vi "ExampleAppAssembler.vi"() -> ()   [LabVIEW 2017]
uses:
  <vilib>/ActorFramework/Message Enqueuer/Message Priority.ctl
  <vilib>/gpm_packages/@cs/mva-viewable/Source/IViewable/IViewable/View Position Enum.ctl
  ViewModel/ViewModel/Test Executive Builder ViewModel.lvclass
  C:/Program Files/National Instruments/LabVIEW 2017/vi.lib/gpm_packages/@cs/mva-core/Source/IObserver/IObserver/IObserver.lvclass
  C:/Program Files/National Instruments/LabVIEW 2017/vi.lib/gpm_packages/@cs/mva-viewable/Source/IViewModel/IViewModel/IViewModel.lvclass
  C:/Program Files/National Instruments/LabVIEW 2017/vi.lib/ActorFramework/Actor/Actor.lvclass
  Test Executive Explorer/Test Executive Explorer/Test Executive Explorer.lvclass
  C:/Program Files/National Instruments/LabVIEW 2017/vi.lib/gpm_packages/@cs/file-explorer-extension/Source/File Explorer/File Explorer/File Explorer.lvclass
  <vilib>/gpm_packages/@cs/persistence/source/XML/XML.lvclass
  C:/Program Files/National Instruments/LabVIEW 2017/vi.lib/gpm_packages/@cs/persistence/source/IPersist/IPersist.lvclass
  <vilib>/gpm_packages/@cs/test-executive/Source/Test Executive/TestExecutive/Test Executive.lvclass
  C:/Program Files/National Instruments/LabVIEW 2017/vi.lib/gpm_packages/@cs/test-executive/Source/Test Executive/ITestExecutive/ITest Executive.lvclass
  Test Executive Builder/Test Executive Builder/Test Executive Builder.lvclass
  D:/Test-executive-builder/Source/Test Executive Builder Model/Test Executive Builder Model/Test Executive Builder Model.lvclass
  C:/Program Files/National Instruments/LabVIEW 2017/vi.lib/gpm_packages/@cs/mva-core/Source/IModel/IModel/IModel.lvclass
  Test Executive View/Test Executive View/Test Executive View.lvclass
  D:/Test-executive-builder/Source/Test Executive Builder View/Test Executive Builder View/Test Executive Builder View.lvclass
  <vilib>/gpm_packages/@cs/test-executive/Source/Path Builder/IPath Builder/IPath Builder.lvclass
  Source/Test Executive Builder Dialogs/Boolean Type View/Boolean Type View.lvclass
  D:/Test-executive-builder/Source/Test Executive Builder Dialogs/IAttribute Data Type View/IAttribute Data Type View.lvclass
  Source/Test Executive Builder Dialogs/String Type View/String Type View.lvclass
  Source/Data Type Handler/Test Executive Builder Data Type Handler.lvclass
  Source/Test Executive Builder Dialogs/Float Type View/Float Type View.lvclass
  Source/Test Executive Builder Dialogs/Integer Type View/Integer Type View.lvclass
  Test Executive View/Test Executive Click Interpreter/Test Executive Click Interpreter.lvclass
  D:/Test-executive-builder/Source/Test Executive Builder View/Tree Click Interpreter/Tree Click Interpreter.lvclass
  Source/Test Executive Builder Dialogs/Edit Subroutine Dialog/Subroutine Dialog.lvclass
  D:/Test-executive-builder/Source/Test Executive Builder Dialogs/ITest Executive Builder Dialog/ITest Executive Builder Dialog.lvclass
  Source/Test Executive Builder Dialogs/Test Step Dialog/Test Step Dialog.lvclass
  Source/Test Executive Builder Dialogs/Name Only Dialog/Name Only Dialog.lvclass
  Source/Test Executive Builder Dialogs/Edit Conditional Dialog/Conditional Dialog.lvclass
  Source/Test Executive Builder Dialogs/For Loop Dialog/For Loop Dialog.lvclass
  <vilib>/gpm_packages/@cs/BusMonitor/ListboxBusMonitor/ListboxBusMonitor/ListboxBusMonitor.lvclass/ListboxBusMonitor.ctl
  <vilib>/gpm_packages/@cs/mva-core/Source/MonitoredMediator/MonitoredMediator/MonitoredMediator.lvclass
  C:/Program Files/National Instruments/LabVIEW 2017/vi.lib/gpm_packages/@cs/mva-core/Source/IMediator/IMediator/IMediator.lvclass
  Source/Test Executive Builder Dialogs/TestStep Edit Dialog/TestStep Edit Dialog.lvclass
  Source/Test Executive Builder Dialogs/LimitType/Numeric Limit.lvclass
  <vilib>/gpm_packages/@cs/mva-core/Source/MonitoredMediator/MonitoredMediator/MonitoredMediator.lvclass/MonitoredMediator.ctl
  Source/Test Executive Builder View/Test Executive Builder View/Test Executive Builder View.lvclass/Test Executive Builder View.ctl
  Test Executive Builder/Test Executive Builder/Test Executive Builder.lvclass/Test Executive Builder.ctl
  <vilib>/gpm_packages/@cs/event-logger/Source/Composed Log/LoggerReference/LoggerReference.lvclass/LoggerReference.ctl
  <vilib>/gpm_packages/@cs/mva-core/Source/IObserver/IObserver/IObserver.lvclass/IObserver.ctl
  <vilib>/gpm_packages/@cs/mva-core/Source/IMediator/IMediator/IMediator.lvclass/IMediator.ctl
  <vilib>/gpm_packages/@cs/mva-viewable/Source/IViewModel/IViewModel/IViewModel.lvclass/IViewModel.ctl
  <vilib>/gpm_packages/@cs/mva-viewable/Source/IViewManager/IViewManager Messages/Launch Nested Views Msg/Launch Nested Views Msg.lvclass/Launch Nested Views Msg.ctl
  <vilib>/gpm_packages/@cs/mva-viewable/Source/IViewManager/IViewManager/IViewManager.lvclass/IViewManager.ctl
  <vilib>/gpm_packages/@cs/mva-viewable/Source/IViewable/IViewable Messages/Open Front Panel Msg/Open Front Panel Msg.lvclass/Open Front Panel Msg.ctl
  <vilib>/ActorFramework/Message Enqueuer/Message Enqueuer.lvclass/Message Enqueuer.ctl
  877fe682-8580-42f1-8583-b2cb626bfff3.vi
  09932d9d-5c8c-44ab-ba7d-36897caed799.vi
  <vilib>/gpm_packages/@cs/mva-core/Source/MonitoredMediator/MonitoredMediator/Private Write BusMonitors.vi
  09932d9d-5c8c-44ab-ba7d-36897caed799.vi/f8c87f9e-9bfc-4d6a-96d5-b886982e97e1.vi
  <vilib>/gpm_packages/@cs/mva-core/Source/IObserver/IObserver/Configure Observer Logging.vi
  <vilib>/gpm_packages/@cs/mva-viewable/Source/IViewModel/IViewModel/Write Startup Model-View Configuration.vi
  <vilib>/gpm_packages/@cs/mva-core/Source/IMediator/IMediator/Configure Mediator.vi
  <vilib>/ActorFramework/Message Enqueuer/Enqueue.vi
  <vilib>/gpm_packages/@cs/event-logger/Source/Composed Log/LoggerReference/Return Aggregate Queues.vi
  <vilib>/gpm_packages/@cs/event-logger/Source/Composed Log/LoggerReference/Add Aggregate Log.vi
  09932d9d-5c8c-44ab-ba7d-36897caed799.vi/f8c87f9e-9bfc-4d6a-96d5-b886982e97e1.vi/92d593a0-8633-4b5a-8c3b-4d6589b4a823.vi
  <vilib>/gpm_packages/@cs/mva-viewable/Source/IViewManager/IViewManager Messages/Launch Nested Views Msg/Pack Launch Nested Views Msg.vi
  <vilib>/gpm_packages/@cs/mva-viewable/Source/IViewManager/IViewManager/Write Startup Launch Nested Views Msg.vi
  <vilib>/gpm_packages/@cs/event-logger/Source/Composed Log/LoggerReference/Send Add Sink.vi
  <vilib>/gpm_packages/@cs/event-logger/Source/Text File Sink/Text File Sink.lvclass
  C:/Program Files/National Instruments/LabVIEW 2017/vi.lib/gpm_packages/@cs/event-logger/Source/Composed Log/Log Sink/Log Sink.lvclass
  Source/Test Executive Builder ViewManager/Test Executive Builder ViewManager/Test Executive Builder ViewManager.lvclass
  C:/Program Files/National Instruments/LabVIEW 2017/vi.lib/gpm_packages/@cs/mva-viewable/Source/IViewable/IViewable/IViewable.lvclass
  <vilib>/gpm_packages/@cs/mva-viewable/Source/IViewModel/IViewModel/IViewModel.lvclass
  C:/Program Files/National Instruments/LabVIEW 2017/vi.lib/gpm_packages/@cs/mva-viewable/Source/IViewManager/IViewManager/IViewManager.lvclass
  <vilib>/gpm_packages/@cs/mva-viewable/Source/IViewable/IViewable Messages/Open Front Panel Msg/Open Front Panel Msg.lvclass
  C:/Program Files/National Instruments/LabVIEW 2017/vi.lib/ActorFramework/Message/Message.lvclass
  <vilib>/gpm_packages/@cs/event-logger/Source/Composed Log/Application Logger/Launch Worker Loop.vi
  <vilib>/gpm_packages/@cs/event-logger/Source/Composed Log/LoggerReference/Initialize Logger Instance.vi
  <vilib>/ActorFramework/Message Priority Queue/Priority Enqueue.vi
  <vilib>/gpm_packages/@cs/BusMonitor/ListboxBusMonitor/ListboxBusMonitor/ListboxBusMonitor.lvclass
  <vilib>/gpm_packages/@cs/event-logger/Source/Composed Log/LoggerReference/LoggerReference.lvclass
  <vilib>/gpm_packages/@cs/event-logger/Source/Composed Log/IErrorFormat/IErrorFormat.lvclass
  <vilib>/gpm_packages/@cs/event-logger/Source/Composed Log/Log Sink/Log Sink.lvclass
  <vilib>/gpm_packages/@cs/mva-viewable/Source/IViewable/IApplicationStyle/IApplicationStyle.lvclass
  <vilib>/gpm_packages/@cs/mva-viewable/Source/IViewManager/IViewManager Messages/Launch Nested Views Msg/Launch Nested Views Msg.lvclass
  <vilib>/ActorFramework/Actor/Actor.lvclass
  <vilib>/ActorFramework/Message Enqueuer/Message Enqueuer.lvclass
  <vilib>/gpm_packages/@cs/mva-viewable/Source/IViewable/IViewable/IViewable.lvclass
  Source/Test Executive Builder Model/Test Executive Builder Model/Test Executive Builder Model.lvclass
  Source/Test Executive Builder View/Test Executive Builder View/Test Executive Builder View.lvclass
panel:
  out "error out":errorcluster
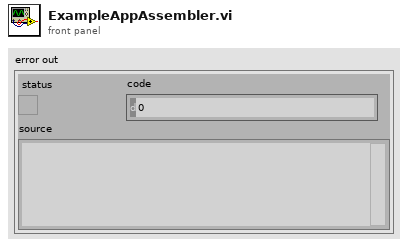
[diagram p1: front panel]
types:
  T1 = typedef "IViewable.lvlib/IViewable.lvclass/View Position Enum.ctl" = enum16{"Centered", "Maximized", "Minimized", "Custom", "Unchanged"}
  T2 = typedef "Actor Framework.lvlib/Message Enqueuer.lvclass/Message Priority.ctl" = enum16{"Low", "Normal", "High"}
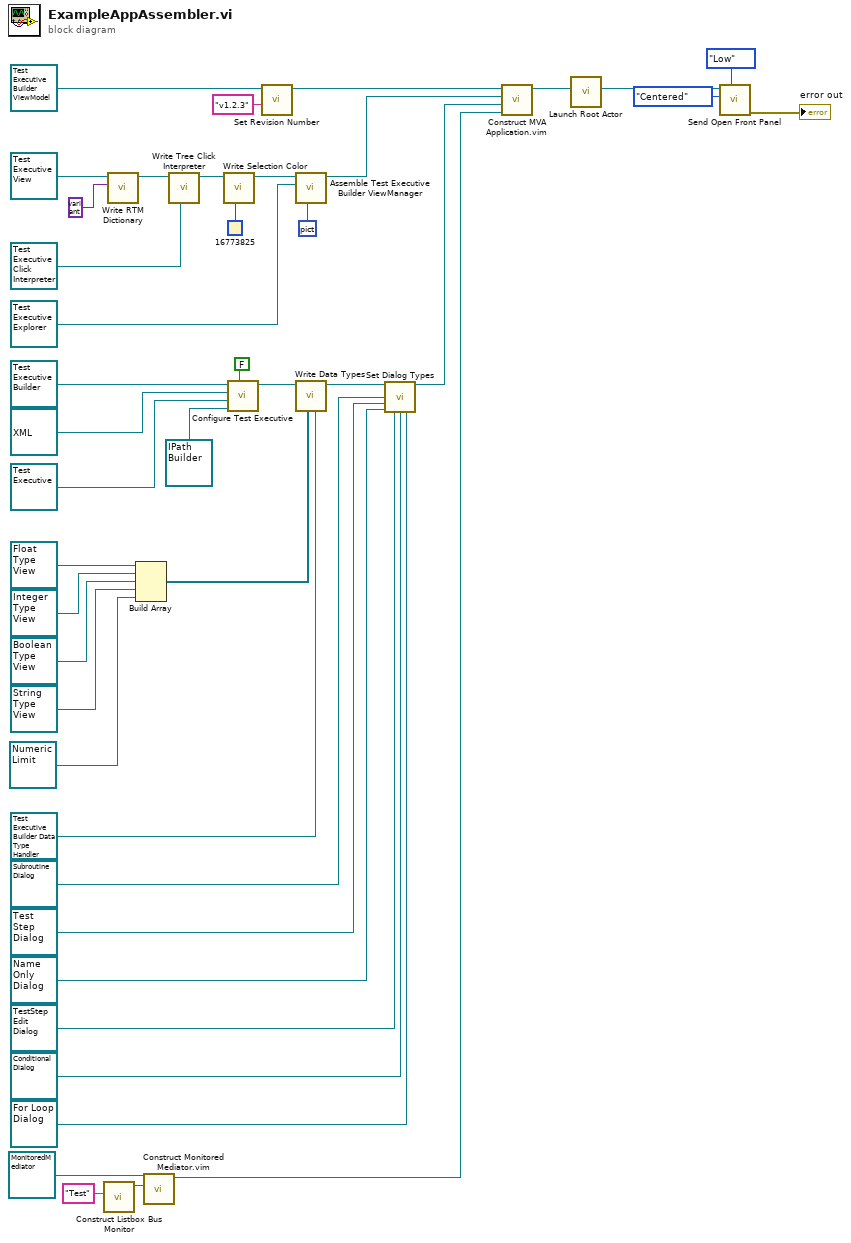
[diagram p0: block diagram]
diagram:
  n1 = call <vilib>:"Construct Listbox Bus Monitor.vi"("Show Panel Boolean Name"="Test") -> ("ListboxBusMonitor out"=w9:refnum<class "ListboxBusMonitor.lvclass">)  [unwired: 10 in]
  n2 = call "Write RTM Dictionary.vi"("RTM Dictionary"=variant, "Test Executive Builder View in"=refnum<class "Test Executive View.lvclass"> refnum ("TestApplication.lvlib:Test Executive View.lvlib:Test Executive View.lvclass")) -> ("Test Executive Builder View out"=w32:refnum<class "Test Executive View.lvclass">)  [unwired: 9 in]
  n3 = Build Array(refnum<class "Float Type View.lvclass"> refnum ("Float Type View.lvclass"), refnum<class "Integer Type View.lvclass"> refnum ("Integer Type View.lvclass"), refnum<class "Boolean Type View.lvclass"> refnum ("Boolean Type View.lvclass"), refnum<class "String Type View.lvclass"> refnum ("String Type View.lvclass"), refnum<class "Numeric Limit.lvclass"> refnum ("Numeric Limit.lvclass")) -> (w22:refnum<class "IAttribute Data Type View.lvclass">[])
  n4 = call "Construct Monitored Mediator.vim"("Startup Bus Monitor(s)"=w9, "MonitoredMediator in"=refnum<class "MonitoredMediator.lvclass"> refnum ("MonitoredMediator.lvlib:MonitoredMediator.lvclass")) -> ("MonitoredMediator out"=w8:refnum<class "MonitoredMediator.lvclass">)  [unwired: 9 in]
  n5 = call "Write Tree Click Interpreter.vi"("Tree Click Interpreter"=refnum<class "Test Executive Click Interpreter.lvclass"> refnum ("Test Executive Click Interpreter.lvclass"), "Test Executive Builder View in"=w32) -> ("Test Executive Builder View out"=w30:refnum<class "Test Executive View.lvclass">)  [unwired: 9 in]
  n6 = call "Write Selection Color.vi"("Selection Color"=u32 16773825, "Test Executive Builder View in"=w30) -> ("Test Executive Builder View out"=w29:refnum<class "Test Executive View.lvclass">)  [unwired: 9 in]
  n7 = call "Configure Test Executive.vi"("Show IDs?"=FALSE, "Path Builder Type"=refnum<class "IPath Builder.lvclass"> refnum, "Test Executive Type"=refnum<class "Test Executive.lvclass"> refnum ("Test Executive.lvlib:Test Executive.lvclass"), "Persistence Type"=refnum<class "XML.lvclass"> refnum ("XML.lvlib:XML.lvclass"), "Test Executive Builder Model in"=refnum<class "Test Executive Builder.lvclass"> refnum ("TestApplication.lvlib:Test Executive Builder.lvlib:Test Executive Builder.lvclass")) -> ("Test Executive Builder Model out"=w25:refnum<class "Test Executive Builder.lvclass">)  [unwired: 6 in]
  n8 = call "Set Revision Number.vi"("Version"="v1.2.3", "Test Executive Builder ViewModel in"=refnum<class "Test Executive Builder ViewModel.lvclass"> refnum ("ViewModelo.lvlib:ViewModel.lvclass")) -> ("Test Executive Builder ViewModel out"=w7:refnum<class "Test Executive Builder ViewModel.lvclass">)  [unwired: 9 in]
  n9 = call "Assemble Test Executive Builder ViewManager.vi"("Dirty Dot True"=picture bytes[830] ("new picture"), "File Explorer View"=refnum<class "Test Executive Explorer.lvclass"> refnum ("TestApplication.lvlib:Test Executive Explorer.lvlib:Test Executive Explorer.lvclass"), "Test Executive Builder View"=w29) -> ("Test Executive Builder ViewManager out"=w6:refnum<class "Test Executive Builder ViewManager.lvclass">)  [unwired: 8 in]
  n10 = call "Write Data Types.vi"("Data Type Handler"=refnum<class "Test Executive Builder Data Type Handler.lvclass"> refnum ("Test Executive Builder Data Type Handler.lvclass"), "Data Type Views"=w22, "Test Executive Builder in"=w25) -> ("Test Executive Builder out"=w15:refnum<class "Test Executive Builder.lvclass">)  [unwired: 8 in]
  n11 = call "Set Dialog Types.vi"("Test Executive Builder in"=w15, "Subroutine Dialog Type"=refnum<class "Subroutine Dialog.lvclass"> refnum ("Subroutine Dialog.lvclass"), "Test Step Dialog Type"=refnum<class "Test Step Dialog.lvclass"> refnum ("Test Step Dialog.lvclass"), "Name Only Dialog Type"=refnum<class "Name Only Dialog.lvclass"> refnum ("Name Only Dialog.lvclass"), "Sequence Dialog Type"=refnum<class "TestStep Edit Dialog.lvclass"> refnum ("TestStep Edit Dialog.lvclass"), "Conditional Dialog Type"=refnum<class "Conditional Dialog.lvclass"> refnum ("Conditional Dialog.lvclass"), "For Loop Dialog Type"=refnum<class "For Loop Dialog.lvclass"> refnum ("For Loop Dialog.lvclass")) -> ("Test Executive Builder out"=w5:refnum<class "Test Executive Builder.lvclass">)  [unwired: 8 in]
  n12 = call "Construct MVA Application.vim"("Mediator Type"=w8, "Model Type"=w5, "Startup View Configuration"=w6, "IViewModel In"=w7) -> ("IViewModel Out"=w43:refnum<class "Test Executive Builder ViewModel.lvclass">)  [unwired: 7 in]
  n13 = call <vilib>:"Launch Root Actor.vi"("Actor"=w43) -> ("Actor's Enqueuer"=w42:refnum<class "Message Enqueuer.lvclass">)  [unwired: 9 in, 1 out]
  n14 = call <vilib>:"Send Open Front Panel.vi"("Message Priority (Normal)"=Message_Priority."Low", "Position"=View_Position_Enum."Centered", "Message Enqueuer"=w42) -> ("error out"=→"error out":errorcluster)  [unwired: 7 in, 1 out]
